vi "LV to ITX  Graph.vi"() -> ()   [LabVIEW 2011]
panel:
  in  "Tab":T1(tab)
  in  "XY Graph":cluster{dbl, dbl}[](graph)
  in  "XY Graph 3":cluster{dbl[], dbl[]}[](graph)
  in  "Intensity Graph":dbl[][](graph)
  in  "Path":path
  in  "filename":string
  in  "open file in Igor?":bool
  # "Igor:\n\\S = superscript\n\\B = subscript\n\\M = normal\n\nexample:\nV\\MS\\B = \"V_S\""
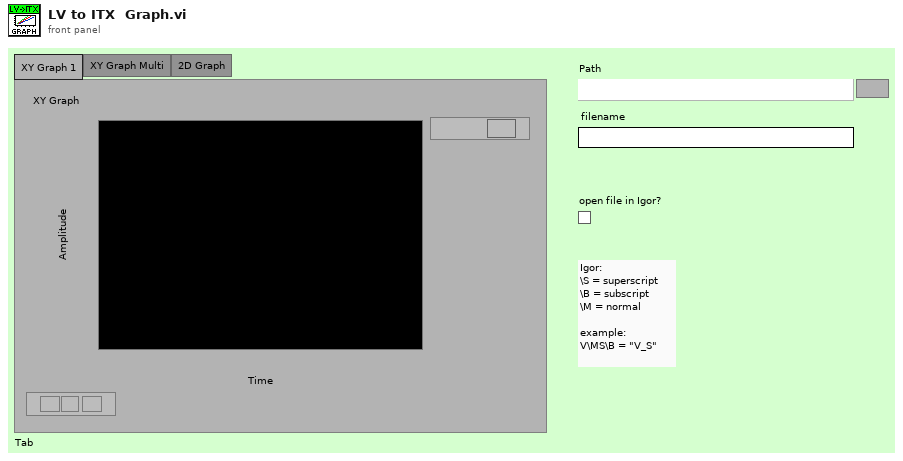
[diagram p1: front panel]
types:
  T1 = enum32{"XY Graph 1", "XY Graph Multi", "2D Graph"}
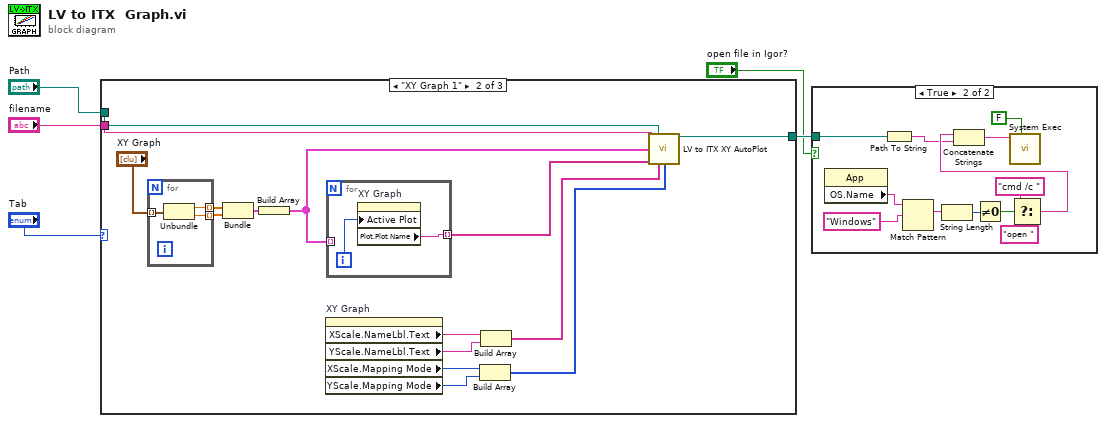
[diagram p0: block diagram]
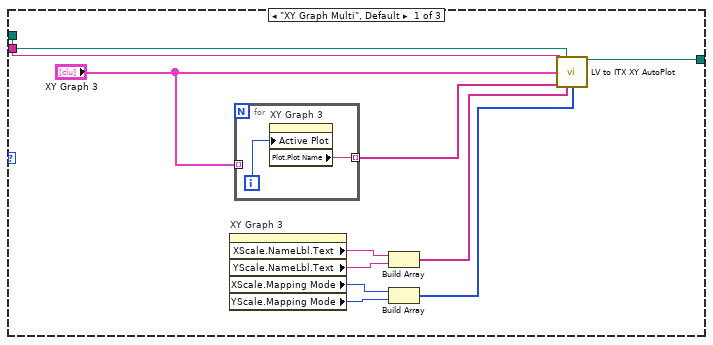
[diagram p3: hidden frame]
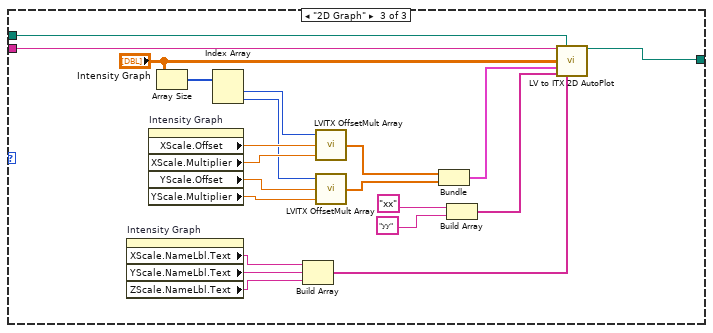
[diagram p4: hidden frame]
diagram:
  n1 = case shown="\"XY Graph 1\"" "Tab" {
    tunnel: "Path" -> [w16 w33 w39]
    tunnel: "filename" -> [w15 w32 w59]
    tunnel: [w11 w31 w46] -> w3
    frame "XY Graph Multi", Default {
      n2 = property on="XY Graph 3" class="XYGraph (strict)"() -> ("XScale.NameLbl.Text"=w13:string, "YScale.NameLbl.Text"=w12:string, "XScale.Mapping Mode"=w8:u8, "YScale.Mapping Mode"=w7:u8)  [unwired: 2 in, 2 out]
      n3 = for {
        tunnel: "XY Graph 3" -> [_] mode=indexing
        tunnel: [w17] -> w10 mode=indexing
        i -> [w18]
        n4 = property on="XY Graph 3" class="XYGraph (strict)"("Active Plot"=w18) -> ("Plot.Plot Name"=w17:string)  [unwired: 2 in, 2 out]
      }
      n5 = Build Array(w13, w12) -> (w9:string[])
      n6 = Build Array(w8, w7) -> (w6:u8[])
      n7 = call "LV to ITX XY AutoPlot.vi"("filename"=w15, "path"=w16, "XY Array"="XY Graph 3", "wavenames (.Vx, etc)"=w10, "X,Y Labels"=w9, "X,Y Log"=w6) -> ("file"=w11:path)  [unwired: 9 in]
    }
    frame "XY Graph 1" {
      n8 = for {
        tunnel: "XY Graph" -> [w36] mode=indexing
        tunnel: [w35] -> w28 mode=indexing
        tunnel: [w34] -> w27 mode=indexing
        n9 = Unbundle(w36) -> (w35:dbl, w34:dbl)
      }
      n10 = Bundle(w28, w27) -> (w26:cluster{dbl[], dbl[]})  [unwired: 1 in]
      n11 = Build Array(w26) -> (w25:cluster{dbl[], dbl[]}[])
      n12 = property on="XY Graph" class="XYGraph (strict)"() -> ("XScale.NameLbl.Text"=w24:string, "YScale.NameLbl.Text"=w23:string, "XScale.Mapping Mode"=w22:u8, "YScale.Mapping Mode"=w21:u8)  [unwired: 2 in, 2 out]
      n13 = for {
        tunnel: w25 -> [_] mode=indexing
        tunnel: [w37] -> w30 mode=indexing
        i -> [w38]
        n14 = property on="XY Graph" class="XYGraph (strict)"("Active Plot"=w38) -> ("Plot.Plot Name"=w37:string)  [unwired: 2 in, 2 out]
      }
      n15 = Build Array(w22, w21) -> (w19:u8[])
      n16 = Build Array(w24, w23) -> (w20:string[])
      n17 = call "LV to ITX XY AutoPlot.vi"("filename"=w32, "path"=w33, "XY Array"=w25, "wavenames (.Vx, etc)"=w30, "X,Y Labels"=w20, "X,Y Log"=w19) -> ("file"=w31:path)  [unwired: 9 in]
    }
    frame "2D Graph" {
      n18 = property on="Intensity Graph" class="IntGraph (strict)"() -> ("XScale.NameLbl.Text"=w48:string, "YScale.NameLbl.Text"=w47:string, "ZScale.NameLbl.Text"=w57:string)  [unwired: 2 in, 2 out]
      n19 = property on="Intensity Graph" class="IntGraph (strict)"() -> ("XScale.Offset"=w54:dbl, "XScale.Multiplier"=w53:dbl, "YScale.Offset"=w51:dbl, "YScale.Multiplier"=w50:dbl)  [unwired: 2 in, 2 out]
      n20 = Array Size(array="Intensity Graph") -> (size(s)=w55:i32[])
      n21 = Index Array(array=w55) -> (element #1=w52:i32, element #2=w40:i32)  [unwired: 2 in]
      n22 = Build Array(w48, w47, w57) -> (w58:string[])
      n23 = call "LVITX OffsetMult Array.vi"("XScale.Multiplier"=w53, "XScale.Offset"=w54, "Numeric"=w52) -> ("Array"=w44:dbl[])
      n24 = call "LVITX OffsetMult Array.vi"("XScale.Multiplier"=w50, "XScale.Offset"=w51, "Numeric"=w40) -> ("Array"=w45:dbl[])
      n25 = Bundle("Array"=w44, "Array"=w45) -> (w49:cluster{"Array":dbl[], "Array":dbl[]})  [unwired: 1 in]
      n26 = Build Array("xx" ("X Scale.Name Label.Text"), "yy" ("X Scale.Name Label.Text")) -> (w43:string[])
      n27 = call "LV to ITX 2D AutoPlot.vi"("filename"=w59, "path"=w39, "2D Array"="Intensity Graph", "X, Y Arrays"=w49, "X, Y wavenames"=w43, "X,Y,Z Labels"=w58) -> ("file"=w46:path)  [unwired: 9 in]
    }
  }
  n28 = case shown="True" "open file in Igor?" {
    tunnel: w3 -> [_ w63]
    frame False {
    }
    frame True {
      n29 = property class="App"() -> ("OS.Name"=w64:string)  [unwired: 2 in, 2 out]
      n30 = Path To String(path=w63) -> (string=w60:string)
      n31 = Match Pattern(string=w64, regular expression="Windows") -> (match substring=w70:string)  [unwired: 1 in, 3 out]
      n32 = String Length(string=w70) -> (length=w69:i32)
      n33 = Not Equal To 0?(x=w69) -> (x != 0?=w67:bool)
      n34 = Select(t="cmd /c ", s=w67, f="open ") -> (s? t:f=w62:string)
      n35 = Concatenate Strings(w62, w60) -> (w71:string)
      n36 = call <vilib>:"System Exec.vi"("wait until completion? (T)"=FALSE, "command line"=w71) -> ()  [unwired: 6 in, 4 out]
    }
  }
